vi "VerifyPassword.vi"(7 "LabVIEW Web Service Request":refnum<class "Web Request.lvclass">) -> ()   [LabVIEW 2013]
uses:
  <vilib>/wsapi/Web Request.lvclass
panel:
  # "Use the Web Service Request input terminal to call the VIs on the Web Services palette. Do not remove it from the connector pane unless you don't need access to the palette."
  # "Each additional control wired to the connector pane will be available as an input in the URL. To include an indicator in terminal-mode output (the default setting), it must also be wired to the connector pane."
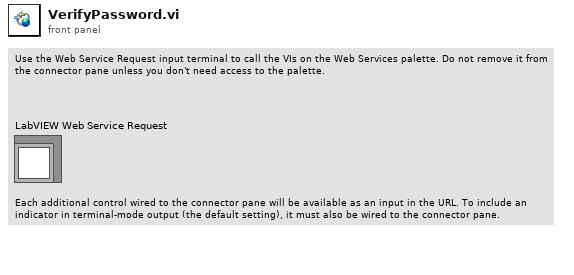
[diagram p1: front panel]
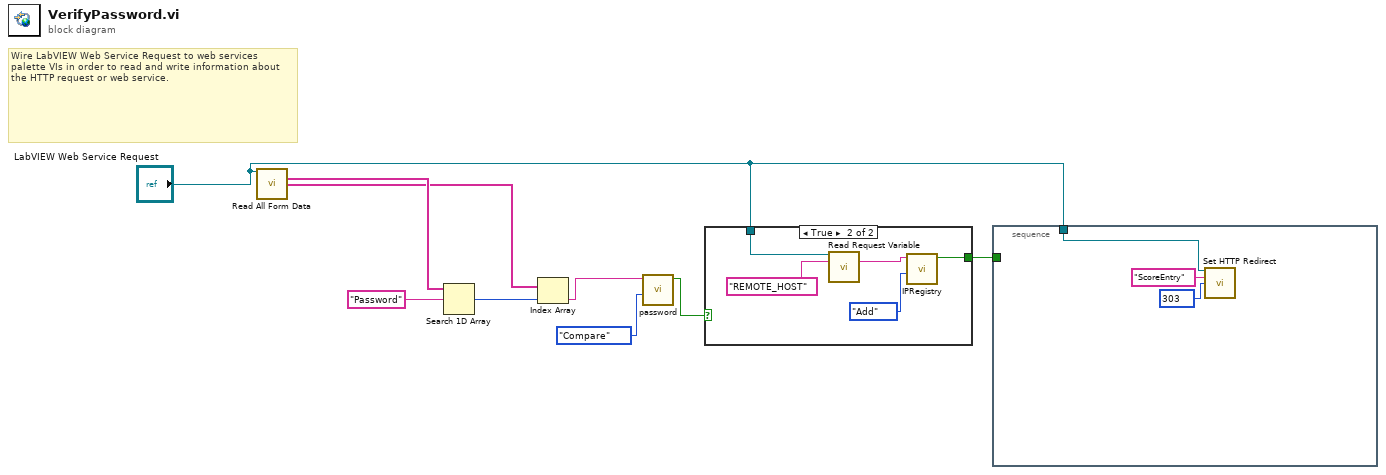
[diagram p0: block diagram]
diagram:
  # "Wire LabVIEW Web Service Request to web services palette VIs in order to read and write information about the HTTP request or web service."
  n1 = call <vilib>:"Read All Form Data.vi"("LabVIEW Web Service Request"="LabVIEW Web Service Request") -> ("Key"=w7:string[], "Value"=w6:string[])  [unwired: 10 in, 3 out]
  n2 = Search 1D Array(1D array=w7, element="Password") -> (index of element=w8:i32)  [unwired: 1 in]
  n3 = Index Array(array=w6, index=w8) -> (element=w5:string)
  n4 = call "password.vi"("Action"=enum16{"Compare", "Set"}."Compare", "password"=w5) -> ("Success?"=w3:bool)  [unwired: 9 in]
  n5 = case shown="True" w3 {
    selector: w3 -> [w10 _]
    tunnel: "LabVIEW Web Service Request" -> [_ w14]
    tunnel: [w10 w11] -> w2
    frame False {
    }
    frame True {
      n6 = call <vilib>:"Read Request Variable.vi"("LabVIEW Web Service Request"=w14, "variable name"="REMOTE_HOST") -> ("value"=w12:string)  [unwired: 11 in, 2 out]
      n7 = call "IPRegistry.vi"("Action"=enum16{"Flush All", "Lookup", "Add"}."Add", "IP Address"=w12) -> ("Success"=w11:bool)  [unwired: 8 in, 1 out]
    }
  }
  n8 = stacked-sequence {
    tunnel: w2 -> [_]
    tunnel: "LabVIEW Web Service Request" -> [w16]
    frame #0 {
      w17 = 303 items=["100"=100, "101"=101, "200"=200, "201"=201, "202"=202, "203"=203, "204"=204, "205"=205, "206"=206, "300"=300, "301"=301, "302"=302, "303"=303, "304"=304, "305"=305, "306"=306, "307"=307, "400"=400, "401"=401, "402"=402, "403"=403, "404"=404, "405"=405, "406"=406, "407"=407, "408"=408, "409"=409, "410"=410, "411"=411, "412"=412, "413"=413, "414"=414, "415"=415, "416"=416, "417"=417, "500"=500, "501"=501, "502"=502, "503"=503, "504"=504, "505"=505] ("response code (307)")
      n9 = call <vilib>:"Set HTTP Redirect.vi"("LabVIEW Web Service Request"=w16, "redirect URL"="ScoreEntry", "response code (307)"=w17) -> ()  [unwired: 11 in, 2 out]
    }
  }
